vi "Configure Alternating Polarity Resistance Resistivity Test.vi"(5 "Discard Readings Number (3)":i32=3, 6 "Store Readings Number (1)":i32=1, 7 "Alternating Voltage (10)":dbl=10.0, 8 "error in (no error)":errorcluster, 9 "Offset Voltage (0)":dbl, 10 "Alternating Measure Time (15 s)":dbl=15.0, 11 "VISA resource name":refnum<visa-resource-name>) -> (0 "error out":errorcluster, 3 "VISA resource name out":refnum<visa-resource-name>)   [LabVIEW 2020, in "Keithley 6517.lvlib"]
doc: "Sets the alternating polarity resistance resistivity test.\n\nNote:\nCall <b> Configure Test Sequence.vi </b> first to arm and configures the test sequence.\n\nThis VI is <B>NOT</B> compatible with model <B>6514</B>."
uses:
  <instrlib>/Keithley 6517/Keithley 6517.lvlib
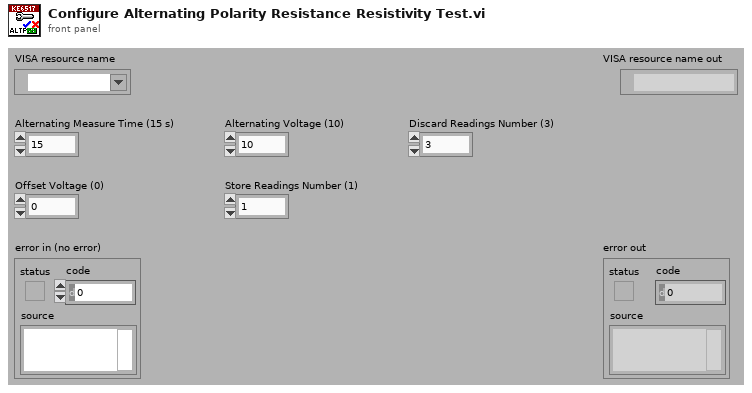
[diagram p1: front panel]
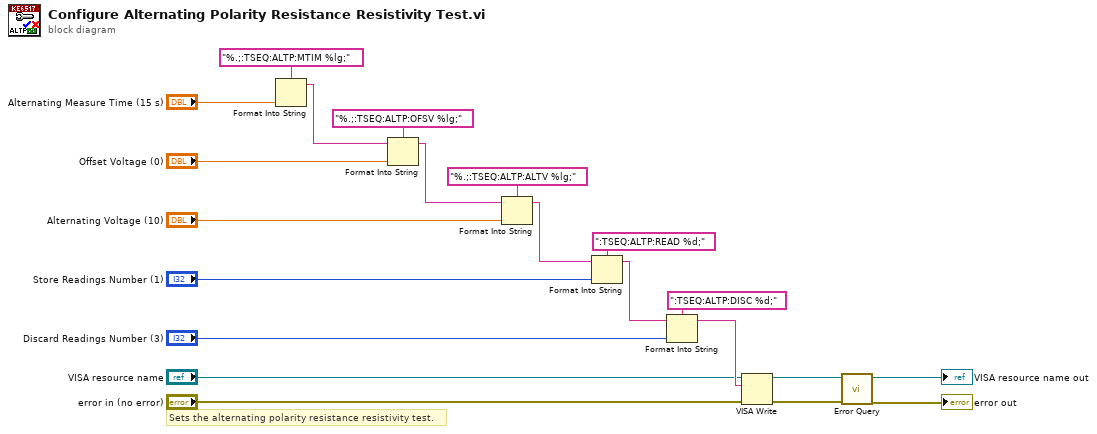
[diagram p0: block diagram]
diagram:
  # "Sets the alternating polarity resistance resistivity test."
  n1 = Format Into String(format string="%.;:TSEQ:ALTP:MTIM %lg;", "Alternating Measure Time (15 s)") -> (resulting string=w19:string)  [unwired: 2 in, 1 out]
  n2 = Format Into String(format string="%.;:TSEQ:ALTP:OFSV %lg;", initial string=w19, "Offset Voltage (0)") -> (resulting string=w16:string)  [unwired: 1 in, 1 out]
  n3 = Format Into String(format string="%.;:TSEQ:ALTP:ALTV %lg;", initial string=w16, "Alternating Voltage (10)") -> (resulting string=w13:string)  [unwired: 1 in, 1 out]
  n4 = Format Into String(format string=":TSEQ:ALTP:READ %d;", initial string=w13, "Store Readings Number (1)") -> (resulting string=w10:string)  [unwired: 1 in, 1 out]
  n5 = Format Into String(format string=":TSEQ:ALTP:DISC %d;", initial string=w10, "Discard Readings Number (3)") -> (resulting string=w7:string)  [unwired: 1 in, 1 out]
  n6 = VISA Write(VISA resource name="VISA resource name", write buffer=w7, error in (no error)="error in (no error)") -> (VISA resource name out=w4:refnum<visa-resource-name>, error out=w3:errorcluster)  [unwired: 1 out]
  n7 = call <instrlib>:"Error Query.vi"("error in (no error)"=w3, "VISA resource name"=w4) -> ("error out"=→"error out":errorcluster, "VISA resource name out"=→"VISA resource name out":refnum<visa-resource-name>)  [unwired: 6 in, 2 out]
